vi "IP_ToDecimalString.vi"(11 "hex string":string) -> (3 "string":string)   [LabVIEW 2020, in "hse-network.lvlib"]
doc: "(v0.2.1b; 2017-08-14 16:44)\n\n\n\n____\nHAMPEL SOFTWARE ENGINEERING v3.8.0 (2023-12-18 14:41)"
uses:
  hse-network.lvlib
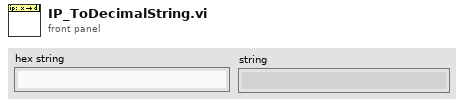
[diagram p1: front panel]
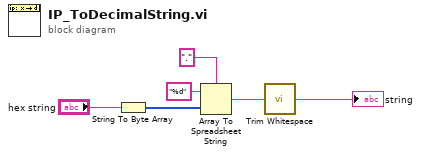
[diagram p0: block diagram]
diagram:
  n1 = String To Byte Array(string="hex string") -> (unsigned byte array=w1:u8[])
  n2 = Array To Spreadsheet String(delimiter (Tab)=".", array=w1, 3:"%d" ("format string")) -> (spreadsheet string=w4:string)
  n3 = call <vilib>:"Trim Whitespace.vi"("string"=w4) -> ("trimmed string"=→"string":string)  [unwired: 1 in]
